vi "CreatePrivateEvents.vi"(10 "error in (no error)":errorcluster) -> (2 "error out":errorcluster, 3 "PrivateEvents":T1)   [LabVIEW 2020, in "CameraTestingProxy.lvlib" / "CameraTestingENI.lvclass"]
uses:
  CameraTestingENI.lvclass
  CameraTestingENI.lvclass/CameraTestingENI.ctl
  CameraTestingApp/ICameraTesting/ICameraTesting/TypeDef/VideoBufferUpdate.ctl
  CameraTestingApp/ICameraTesting/ICameraTesting/ICameraTesting.lvclass
  CameraTestingApp/ICameraTesting/ICameraTesting/TypeDef/StatusRecord.ctl
  CameraTestingApp/ICameraTesting/ICameraTesting/TypeDef/StatusUpdated.ctl
  CameraTestingApp/ICameraTesting/ICameraTesting/TypeDef/VideoOptionsInfo.ctl
  CameraTestingApp/ICameraTesting/ICameraTesting/TypeDef/VideoOptCodesUpdated.ctl
  CameraTestingApp/ICameraTesting/ICameraTesting/TypeDef/ResolutionValReceived.ctl
  CameraTestingApp/ICameraTesting/ICameraTesting/TypeDef/ImgTypeValReceived.ctl
  CameraTestingApp/ICameraTesting/ICameraTesting/TypeDef/FrameRateValReceived.ctl
  Camera/ICamera/ICamera/TypeDef/SnapInfo.ctl
  Camera/ICamera/ICamera/ICamera.lvclass
  CameraTestingApp/ICameraTesting/ICameraTesting/TypeDef/Events.ctl
  <vilib>/ActorFramework/Message Enqueuer/Message Enqueuer.lvclass
  TypeDef/QuitActorEvn.ctl
  TypeDef/CamTestEnqrReceived.ctl
  TypeDef/PrivateEvents.ctl
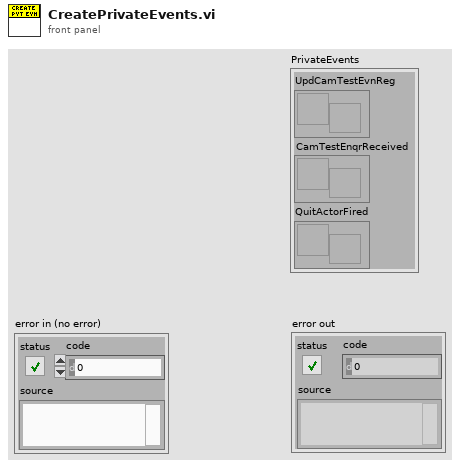
[diagram p1: front panel]
types:
  T1 = typedef "CameraTestingProxy.lvlib/CameraTestingENI.lvclass/PrivateEvents.ctl" = cluster{"UpdCamTestEvnReg":refnum<user-event>, "CamTestEnqrRcv":T2, "QuitActorFired":T3}
  T2 = typedef "CameraTestingProxy.lvlib/CameraTestingENI.lvclass/CamTestEnqrReceived.ctl" = refnum<user-event>
  T3 = typedef "CameraTestingProxy.lvlib/CameraTestingENI.lvclass/QuitActorEvn.ctl" = refnum<user-event>
  T4 = typedef "ICameraTesting.lvlib/ICameraTesting.lvclass/Events.ctl" = cluster{"NewSnapData":refnum<user-event>, "FrameRateValReceived":T5, "ImgTypeValReceived":T6, "ResolutionValReceived":T7, "VideoOptInfoUpdated":T8, "StatusUpdated":T9, "VideoBufferUpdate":T10}
  T5 = typedef "ICameraTesting.lvlib/ICameraTesting.lvclass/FrameRateValReceived.ctl" = refnum<user-event>
  T6 = typedef "ICameraTesting.lvlib/ICameraTesting.lvclass/ImgTypeValReceived.ctl" = refnum<user-event>
  T7 = typedef "ICameraTesting.lvlib/ICameraTesting.lvclass/ResolutionValReceived.ctl" = refnum<user-event>
  T8 = typedef "ICameraTesting.lvlib/ICameraTesting.lvclass/VideoOptCodesUpdated.ctl" = refnum<user-event>
  T9 = typedef "ICameraTesting.lvlib/ICameraTesting.lvclass/StatusUpdated.ctl" = refnum<user-event>
  T10 = typedef "ICameraTesting.lvlib/ICameraTesting.lvclass/VideoBufferUpdate.ctl" = refnum<user-event>
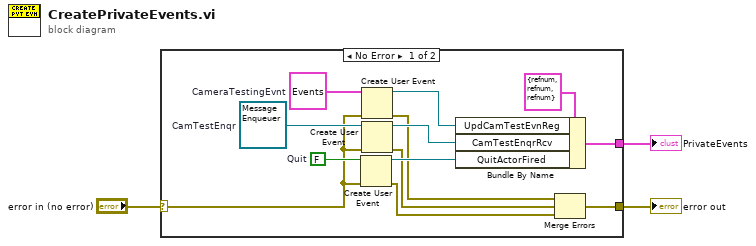
[diagram p0: block diagram]
diagram:
  n1 = case shown="No Error" "error in (no error)" {
    selector: "error in (no error)" -> [w4 w17]
    tunnel: [w9 _] -> w3
    tunnel: [w5 w17] -> w2
    frame No Error {
      w14 = refnum<class "Message Enqueuer.lvclass"> refnum  # CamTestEnqr
      w15 = FALSE  # Quit
      w16 = T4 {"NewSnapData"=refnum, "FrameRateValReceived"=refnum, "ImgTypeValReceived"=refnum, "ResolutionValReceived"=refnum, "VideoOptInfoUpdated"=refnum, "StatusUpdated"=refnum, "VideoBufferUpdate"=refnum}  # CameraTestingEvnt
      n2 = Create User Event(user event datatype=w15, error in=w4) -> (user event=w10:refnum<user-event>, error out=w6:errorcluster)
      n3 = Create User Event(user event datatype=w16, error in=w4) -> (user event=w12:refnum<user-event>, error out=w8:errorcluster)
      n4 = Create User Event(user event datatype=w14, error in=w4) -> (user event=w11:refnum<user-event>, error out=w7:errorcluster)
      n5 = Bundle By Name(cluster=T1 {"UpdCamTestEvnReg"=refnum, "CamTestEnqrRcv"=refnum, "QuitActorFired"=refnum} ("PrivateEvents"), "UpdCamTestEvnReg"=w12, "CamTestEnqrRcv"=w11, "QuitActorFired"=w10) -> (w9:T1)
      n6 = Merge Errors(w8, w7, w6) -> (w5:errorcluster)
    }
    frame Error {
    }
  }
  "PrivateEvents" <- w3
  "error out" <- w2
